vi "SOF and EOF 14443A.vi"(11 "Bit stream in Miller":u8[](array[numeric])=[0, 0, 0, 0, 0, 0, 0, 0, 0, 0, 1, 1]) -> (3 "Bit stream out Miller":u8[](array[numeric]))   [LabVIEW 2019]
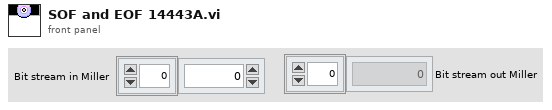
[diagram p1: front panel]
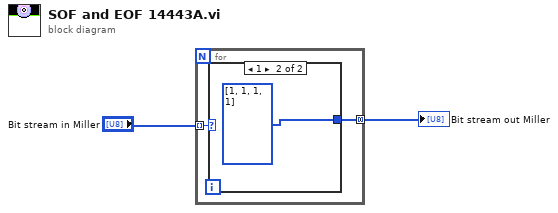
[diagram p0: block diagram]
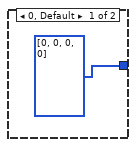
[diagram p2: hidden frame]
diagram:
  n1 = for {
    tunnel: "Bit stream in Miller" -> [w4] mode=indexing
    tunnel: [w3] -> w1 mode=concatenating
    n2 = case shown="1" w4 {
      tunnel: [u8[] [0, 0, 0, 0] ("Bit stream out (NRZ encode)") u8[] [1, 1, 1, 1] ("Bit stream out (NRZ encode)")] -> w3
      frame 0, Default {
      }
      frame 1 {
      }
    }
  }
  "Bit stream out Miller" <- w1
